vi "Convert Error from Boolean False.vi"(7 "Convert to Error Code":T1, 8 "error in (no error)":errorcluster, 10 "Error Message (\"\")":string, 11 "Error Input":bool) -> (0 "error out":errorcluster)   [LabVIEW 2018, in "Scripting.lvlib"]
doc: "Convert an range of Error-Inputs into the Error Code specified. This VI supports converting the following into errors:\n - Error Cluster (with error)\n - Empty Path/Refnum\n - Boolean False\n - Empty Array\n - Empty String"
uses:
  Scripting.lvlib
  Error-Codes.ctl
  Error-Offset.vi
  <vilib>/Utility/error.llb/Error Cluster From Error Code.vi
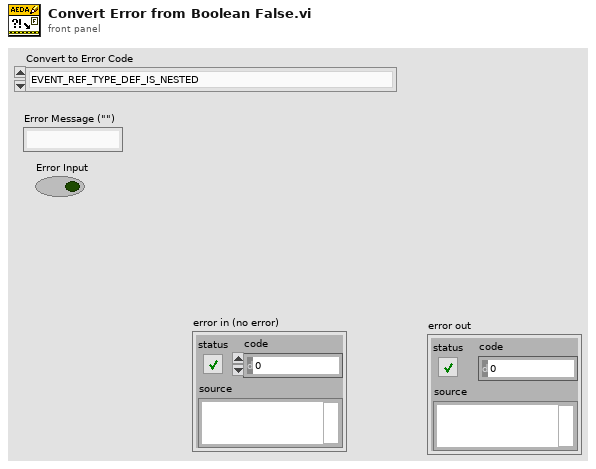
[diagram p1: front panel]
types:
  T1 = typedef "Scripting.lvlib/Error-Codes.ctl" = enum16{"EVENT_REF_TYPE_DEF_IS_NESTED", "EVENT_REF_TYPE_DEF_IS_EMPTY", "EVENT_REF_TYPE_DEF_INCLUDES_NON_REFS", "EVENT_REF_TYPE_INVALID_REPLY_REF", "EVENT_REF_TYPE_REPLY_IS_NOT_TYPE_DEF", "EVENT_REF_TYPE_DEF_IS_NOT_CLUSTER", "EVENT_REF_TYPE_DEF_INVALID_REQ_REPLY_TYPE", "ACTOR_CLASS_PATH_IS_INVALID", "ACTOR_CLASS_LIBRARY_IS_NOT_EDITABLE", "ACTOR_CLASS_CREATE_ENQUEUER_REFS_VI_NOT_FOUND", "MSG_ENQUEUER_REFS_CTL_NOT_FOUND", "ACTOR_CLASS_MAIN_RUN_VI_NOT_FOUND", "ACTOR_CLASS_DESTROY_ENQUEUER_REFS_VI_NOT_FOUND", "CREATE_ENQUEUER_REFS_ERROR_TERMINAL_NOT_FOUND", "CREATE_ENQUEUER_REFS_INVALID_TYPE_DEF", "CREATE_ENQUEUER_REF_NAMEBUNDLER_NOT_FOUND", "CREATE_ENQUEUER_REF_MULTIPLE_NAMEBUNDLERS", "MESSAGES_REF_TYPE_DEF_IS_EMPTY", "MESSAGES_REF_TYPE_DEF_IS_NESTED", "ACTOR_TEMPLATE_CLASS_NOT_FOUND"}
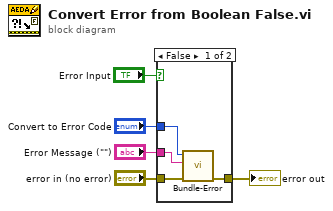
[diagram p0: block diagram]
diagram:
  n1 = case shown="False" "Error Input" {
    tunnel: [w8 w10] -> w2
    tunnel: "error in (no error)" -> [w9 w10]
    tunnel: "Convert to Error Code" -> [w7 _]
    tunnel: "Error Message (\"\")" -> [w6 _]
    frame False {
      n2 = call "Bundle-Error.vi"("error in (no error)"=w9, "error message (\"\")"=w6, "Errors"=w7) -> ("error out"=w8:errorcluster)  [unwired: 8 in]
    }
    frame True {
    }
  }
  "error out" <- w2
